vi "args control name.vi"() -> (3 "args control name":string)   [LabVIEW 2013]
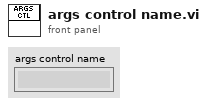
[diagram p1: front panel]
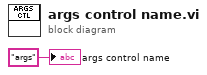
[diagram p0: block diagram]
diagram:
  "args control name" <- "args" ("format string")
